vi "Doğrusalsızlık Sub-VI.vi"() -> ()   [LabVIEW 2015]
uses:
  <vilib>/Utility/file.llb/Read Delimited Spreadsheet (DBL).vi
panel:
  out "Array":dbl[](array[numeric])
  out "N (Difference)":dbl[](array[numeric])
  out "Calculated(mA)":dbl[](array[numeric])
  out "in (kg)":dbl[](array[numeric])
  out "Döngü  Sayısı":i32
  out "Slope":dbl
  out "% max non-linearity value":dbl
  out "max non-linearity value":dbl
  out "x2":sgl
  out "x1":sgl
  out "y2":sgl
  out "y1":sgl
  in  "Ölçme Sayısını Giriniz":i32
  in  "Path":path
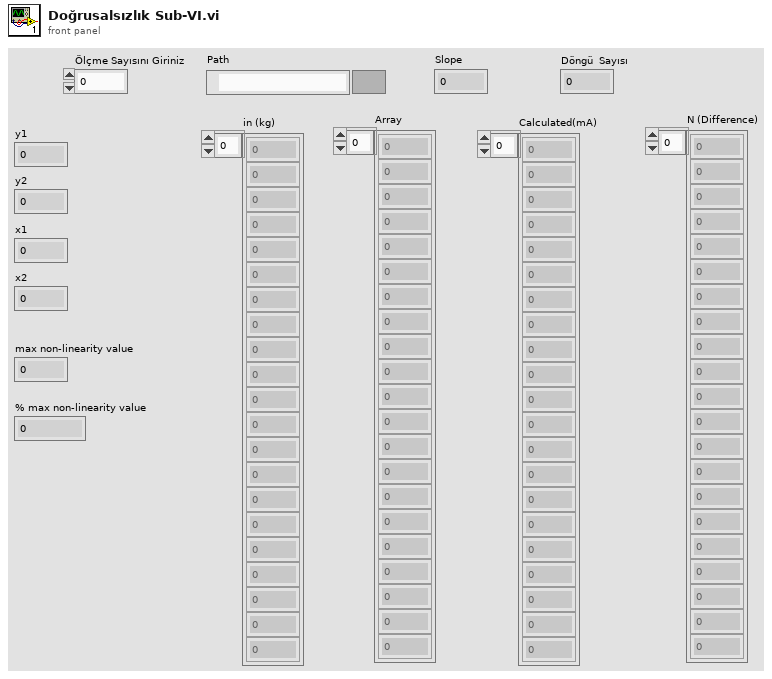
[diagram p1: front panel]
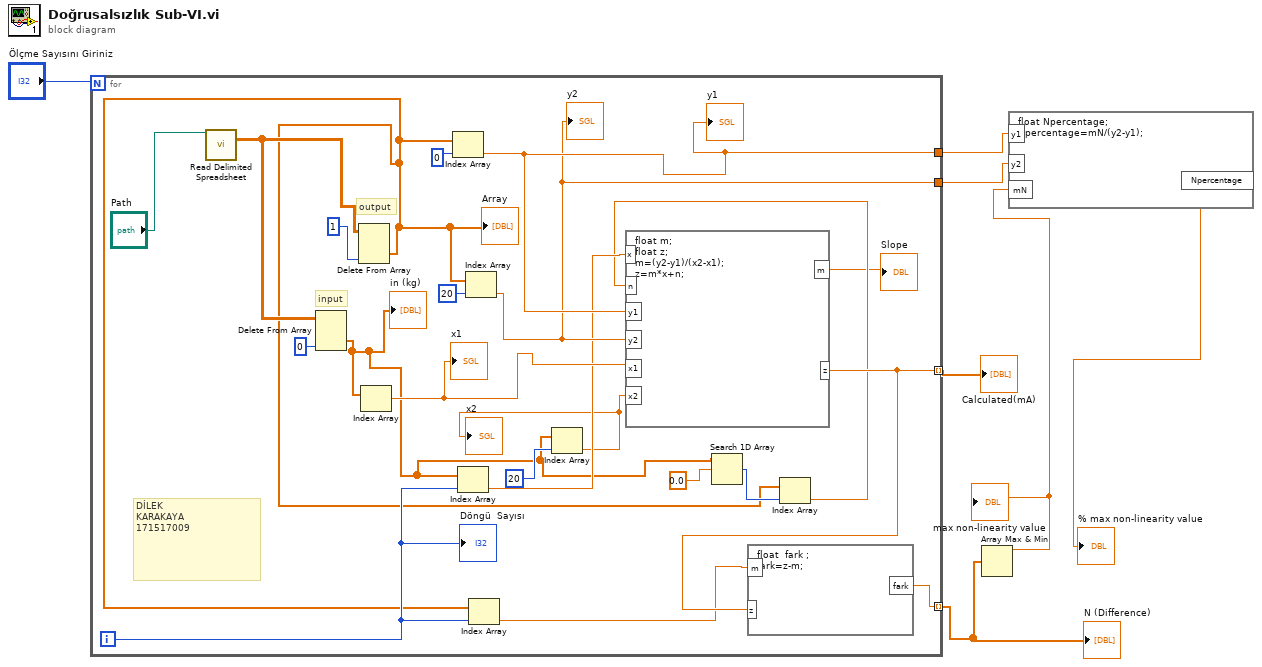
[diagram p0: block diagram]
diagram:
  n1 = for {
    N: "Ölçme Sayısını Giriniz" -> [_]
    tunnel: [w29] -> w1 mode=indexing
    tunnel: [w22] -> w3
    tunnel: [w21] -> w4
    tunnel: [w20] -> w2 mode=indexing
    i -> [w26]
    # "DİLEK \nKARAKAYA\n171517009"
    # "input"
    # "output"
    n2 = call-poly <vilib>:"Read Delimited Spreadsheet.vi"("file path (dialog if empty)"="Path") -> ("all rows"=w10:dbl[][])  [unwired: 9 in, 5 out]
    n3 = Delete From Array(array=w10, index (col)=0 ("disabled index (col)")) -> (deleted portion=w11:dbl[])  [unwired: 2 in, 1 out]
    "in (kg)" <- w11
    n4 = Delete From Array(array=w10, index (col)=1 ("index (row)")) -> (deleted portion=w8:dbl[])  [unwired: 2 in, 1 out]
    "Array" <- w8
    n5 = Index Array(array=w11) -> (element=w25:dbl)  [unwired: 1 in]
    "x1" <- w25
    n6 = Index Array(array=w8, index=0) -> (element=w22:dbl)
    "y1" <- w22
    n7 = Index Array(array=w11, index=w26) -> (element=w17:dbl)
    n8 = Index Array(array=w8, index=20) -> (element=w21:dbl)
    "y2" <- w21
    n9 = Index Array(array=w8, index=w26) -> (element=w19:dbl)
    n10 = Index Array(array=w11, index=20) -> (element=w13:dbl)
    "x2" <- w13
    n11 = Search 1D Array(1D array=w11, element=0.0) -> (index of element=w18:i32)  [unwired: 1 in]
    n12 = Index Array(array=w8, index=w18) -> (element=w16:dbl)
    n13 = formula code="float m;\nfloat z;\nm=(y2-y1)/(x2-x1);\nz=m*x+n;"("x"=w17, "n"=w16, "y1"=w22, "y2"=w21, "x1"=w25, "x2"=w13) -> ("m"=→"Slope":dbl, "z"=w20:dbl)
    n14 = formula code="float  fark ;\nfark=z-m;"("m"=w19, "z"=w20) -> ("fark"=w29:dbl)
    "Döngü  Sayısı" <- w26
  }
  "N (Difference)" <- w1
  "Calculated(mA)" <- w2
  n15 = Array Max & Min(array=w1) -> (max value=w5:dbl)  [unwired: 3 out]
  "max non-linearity value" <- w5
  n16 = formula code="float Npercentage;\nNpercentage=mN/(y2-y1);"("y1"=w3, "y2"=w4, "mN"=w5) -> ("Npercentage"=→"% max non-linearity value":dbl)
